vi "Speed of light V2.vi"(8 "Stop":bool, 10 "Slide":dbl(slide) scale=0.0..100.0, 11 "path":path) -> ()   [LabVIEW 2023]
uses:
  <vilib>/sound2/lvsound2.llb/Sound Output Set Volume (Single).vi
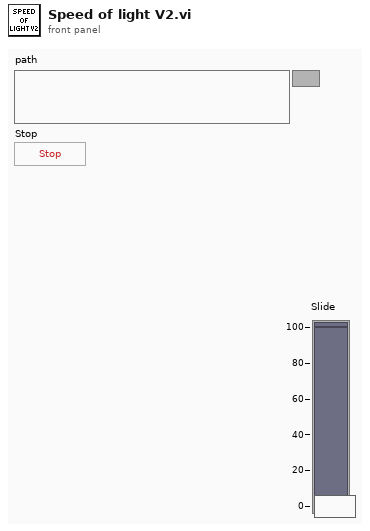
[diagram p1: front panel]
types:
  T1 = typedef "Sound Output Task ID.ctl" = u32
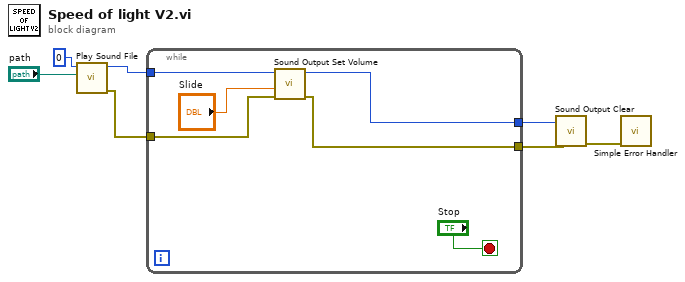
[diagram p0: block diagram]
diagram:
  n1 = call <vilib>:"Play Sound File.vi"("path"="path", "device ID"=u32 0) -> ("error out"=w4:errorcluster, "task ID"=w6:T1)  [unwired: 8 in]
  n2 = while {
    tunnel: w6 -> [w12]
    tunnel: w4 -> [w11]
    tunnel: [w10] -> w3
    tunnel: [w9] -> w1
    stop <- "Stop" stop-if-true
    n3 = call-poly <vilib>:"Sound Output Set Volume.vi"("error in (no error)"=w11, "volume"="Slide", "task ID"=w12) -> ("error out"=w10:errorcluster, "task ID out"=w9:T1)  [unwired: 7 in]
  }
  n4 = call <vilib>:"Sound Output Clear.vi"("error in (no error)"=w3, "task ID"=w1) -> ("error out"=w2:errorcluster)  [unwired: 9 in]
  n5 = call <vilib>:"Simple Error Handler.vi"("error in (no error)"=w2) -> ()  [unwired: 4 in, 5 out]
